vi "array - sorted inexes.vi"(11 "x":dbl[](array[numeric])=[1.0, 5.0, 3.0, 7.0, 0.0]) -> (1 "index array":i32[](array[numeric]), 2 "sorted array":dbl[](array[numeric]))   [LabVIEW 2015]
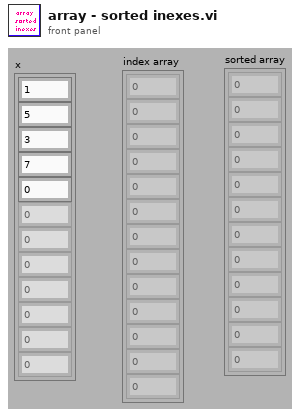
[diagram p1: front panel]
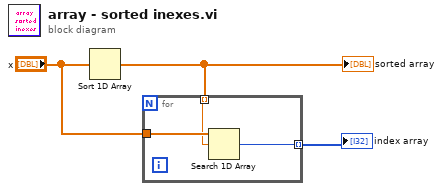
[diagram p0: block diagram]
diagram:
  n1 = Sort 1D Array(array="x") -> (sorted array=w2:dbl[])
  "sorted array" <- w2
  n2 = for {
    tunnel: "x" -> [w6]
    tunnel: w2 -> [w5] mode=indexing
    tunnel: [w4] -> w1 mode=indexing
    n3 = Search 1D Array(1D array=w6, element=w5) -> (index of element=w4:i32)  [unwired: 1 in]
  }
  "index array" <- w1
